vi "WSRealm.vi"(7 "LabVIEW Web Service Request":refnum<class "Web Request.lvclass">) -> ()   [LabVIEW 2013]
doc: "Basic access authentication for any RESTful web service method.\nUsername and password have to be combined to a string \"username:password\" and Base64-encoded."
uses:
  <vilib>/wsapi/Web Request.lvclass
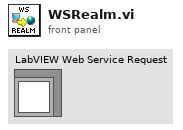
[diagram p1: front panel]
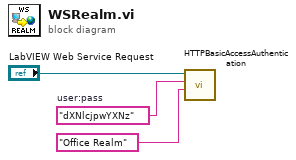
[diagram p0: block diagram]
diagram:
  w1 = "dXNlcjpwYXNz"  # user:pass
  n1 = call "HTTPBasicAccessAuthentication.vi"("Realm"="Office Realm", "Base64 user:pass"=w1, "LabVIEW Web Service Request"="LabVIEW Web Service Request") -> ()  [unwired: 8 in, 1 out]
